vi "Toggle Debug Visible.vi"(6 "ACK":bool, 8 "error in":errorcluster, 11 "Visible?":bool) -> (0 "error out":errorcluster)   [LabVIEW 2015, in "Generic Module Library.lvlib" / "Template G_Module.lvlib"]
uses:
  Template G_Module.lvlib
  Private Controls/Module Message Cluster Components/Message Data Cluster.ctl
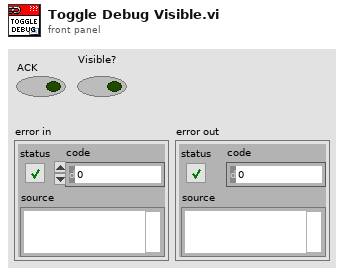
[diagram p1: front panel]
types:
  T1 = typedef "Generic Module Library.lvlib/Template G_Module.lvlib/Message Data Cluster.ctl" = cluster{"Module Action":string, "Message Data":variant}
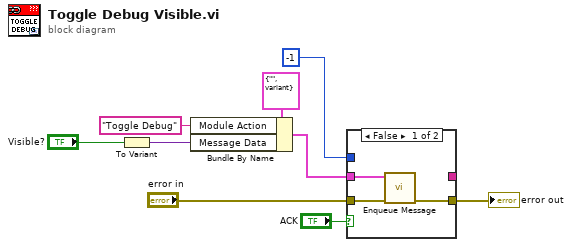
[diagram p0: block diagram]
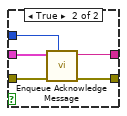
[diagram p2: hidden frame]
diagram:
  n1 = To Variant(anything="Visible?") -> (Variant=w1:variant)
  n2 = Bundle By Name(cluster=T1 {"Module Action"="", "Message Data"=variant} ("Message Data"), "Module Action"="Toggle Debug", "Message Data"=w1) -> (w6:T1)
  n3 = case shown="False" "ACK" {
    tunnel: "error in" -> [w12 w17]
    tunnel: [w11 w16] -> w8
    tunnel: w6 -> [w10 w15]
    tunnel: -1 ("Ack Timeout") -> [_ w14]
    tunnel: [_ w13] -> _
    frame False {
      n4 = call "Enqueue Message.vi"("error in"=w12, "Message Data"=w10) -> ("error out"=w11:errorcluster)  [unwired: 9 in]
    }
    frame True {
      n5 = call "Enqueue Acknowledge Message.vi"("Ack Timeout"=w14, "error in"=w17, "Message Data"=w15) -> ("error out"=w16:errorcluster, "Response Data"=w13:string)  [unwired: 6 in, 1 out]
    }
  }
  "error out" <- w8
